vi "example_temp_monitor_multiqueue.vi"() -> ()   [LabVIEW 2025]
uses:
  <resource>/dialog/BookmarkManager/managers/Default/support/Message Queue/BMark_Message Queue.lvlib
  <resource>/dialog/BookmarkManager/managers/Default/support/User Event - Stop/BMark_User Event - Stop.lvlib
  controls_queue/UI Data.ctl
  Program Files/National Instruments/LabVIEW 2025/examples/Industry Applications/Temperature Monitoring/support/Message Queue/Temp Monitor Message Queue.lvlib
  Program Files/National Instruments/LabVIEW 2025/ProjectTemplates/Source/Core/Continuous Measurement/Logging/Logging Configuration.ctl
  Program Files/National Instruments/LabVIEW 2025/ProjectTemplates/Source/Core/Continuous Measurement/Acquisition/Signal Type.ctl
  Program Files/National Instruments/LabVIEW 2025/ProjectTemplates/Source/Core/Continuous Measurement/Acquisition/Hardware Configuration.ctl
  Program Files/National Instruments/LabVIEW 2025/ProjectTemplates/Source/Core/Continuous Measurement/Settings/Settings.ctl
panel:
  out "Do Something Ref":refnum<vi>
  out "Boolean <Replace Me>":bool
  out "Status":string
  in  "Exit":bool
  in  "Stop":bool
  in  "Settings":bool
  in  "Start":bool
  out "Data":waveform(dbl)[](graph)
  # "Continuous Measurement and Logging (NI-DAQmx)"
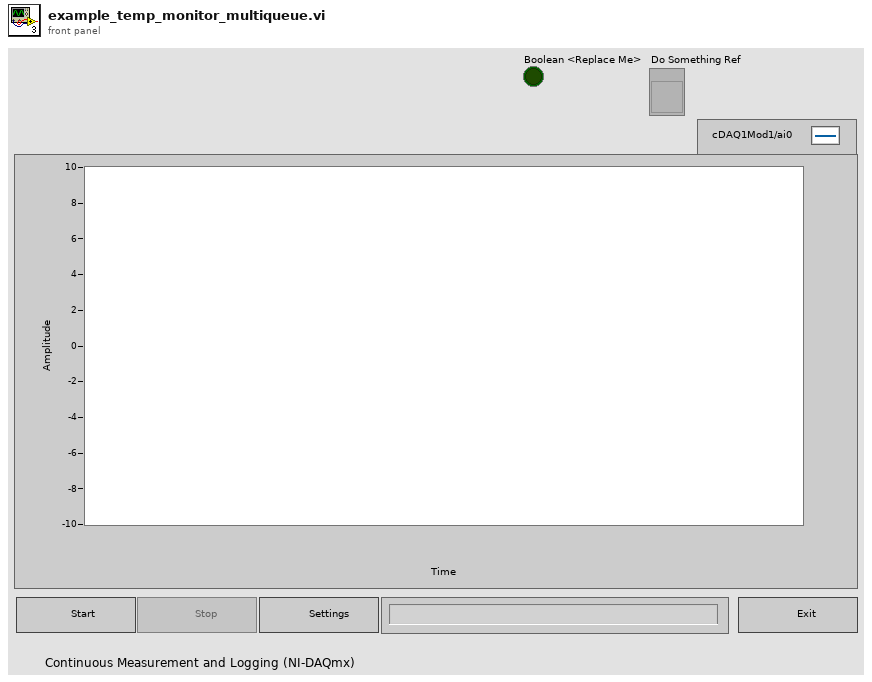
[diagram p1: front panel]
types:
  T1 = typedef "Logging.lvlib/Logging Configuration.ctl" = cluster{"Log File Base Path":path, "TDMS File Reference":refnum<k34>}
  T2 = typedef "Settings.lvlib/Settings.ctl" = cluster{"Hardware Configuration":T3, "Logging Configuration":T1}
  T3 = typedef "Acquisition.lvlib/Hardware Configuration.ctl" = cluster{"HW Refnum <Replace Me>":string, "Signal Type <Replace Me>":T4}
  T4 = typedef "Acquisition.lvlib/Signal Type.ctl" = enum16{"Sine Wave", "Square with Noise"}
  T5 = typedef "UI Data.ctl" = cluster{"Start Ref":refnum<vi>, "Stop Ref":refnum<vi>, "Settings Ref":refnum<vi>, "Exit Ref":refnum<vi>, "Status Ref":refnum<vi>, "Data Ref":refnum<vi>}
  T6 = typedef "Temp Monitor Message Queue.lvlib/All Message Queues.ctl" = cluster{"UI":refnum<queue>, "Acquisition":refnum<queue>}
  T7 = enum16{"open", "open or create", "create or replace", "create", "open (read-only)"}
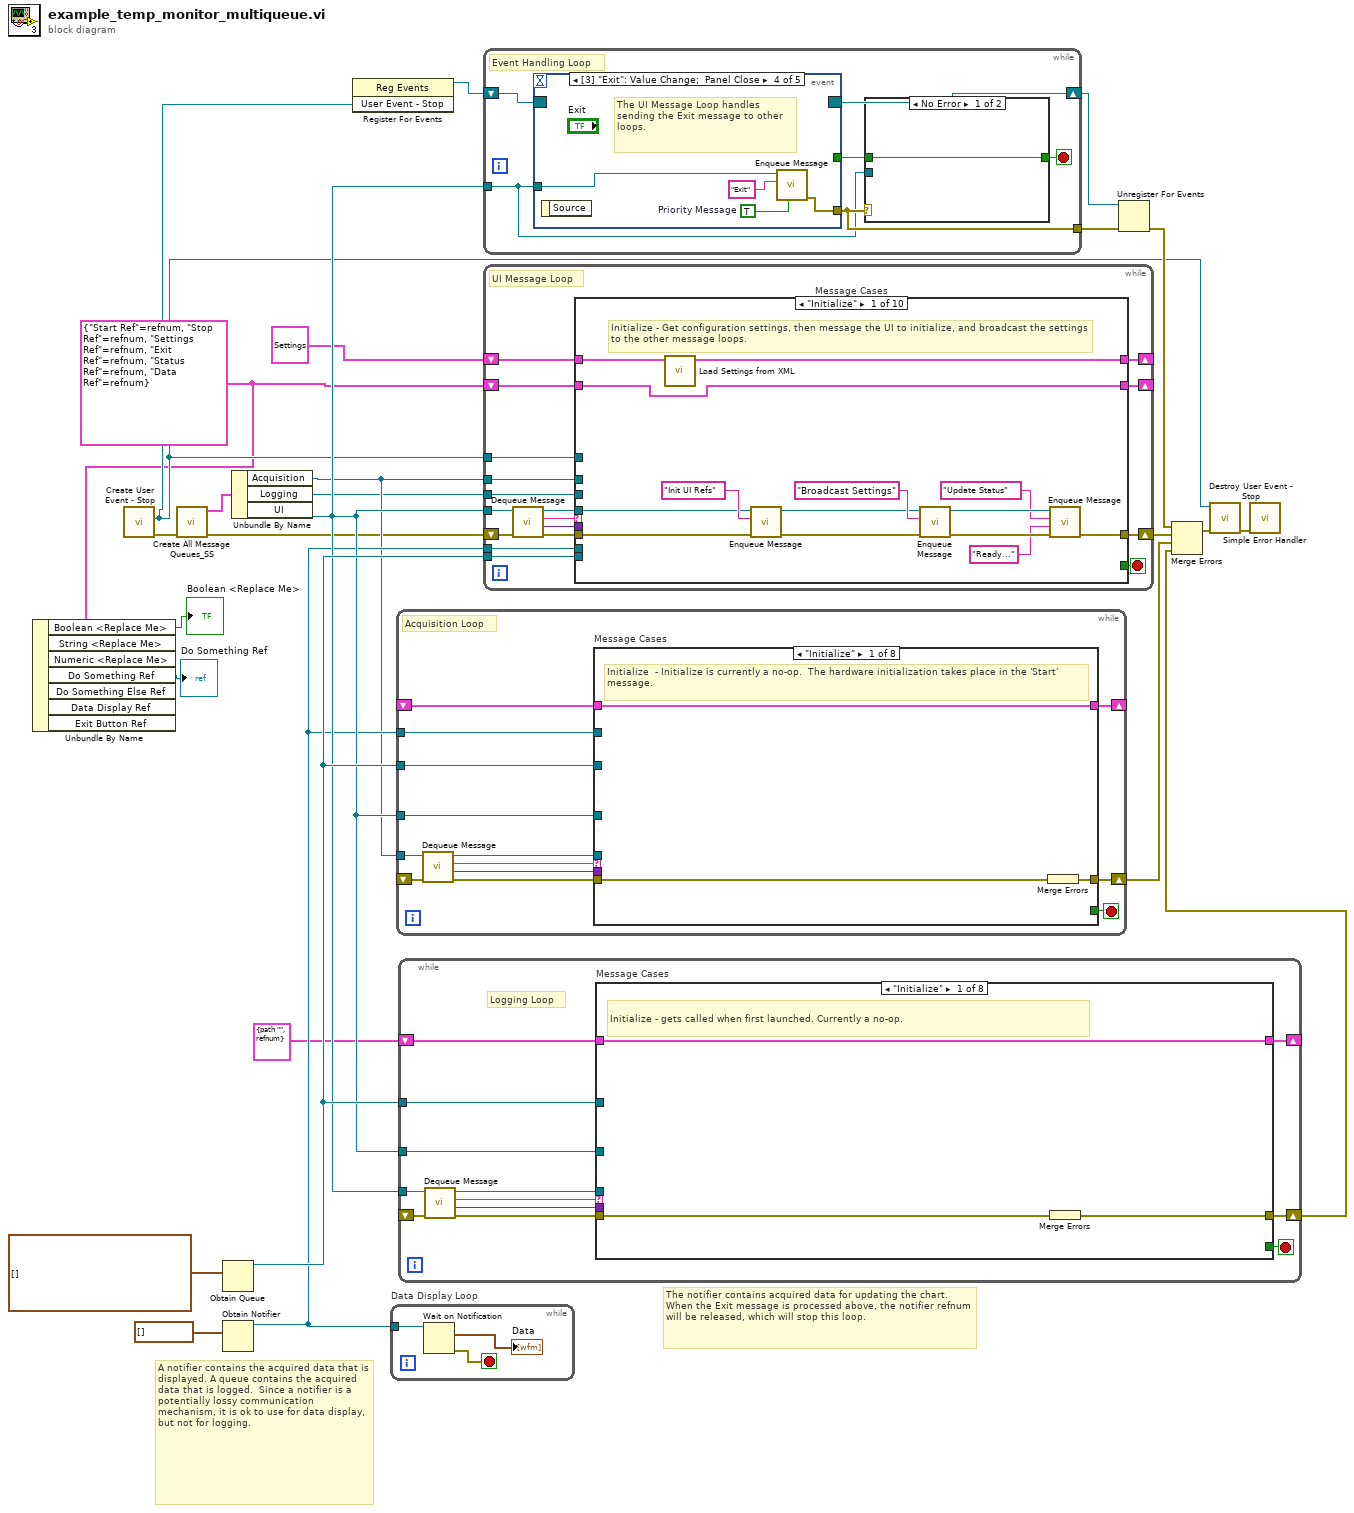
[diagram p0: block diagram]
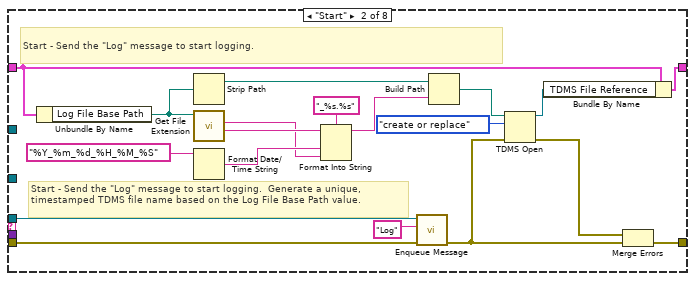
[diagram p2: hidden frame]
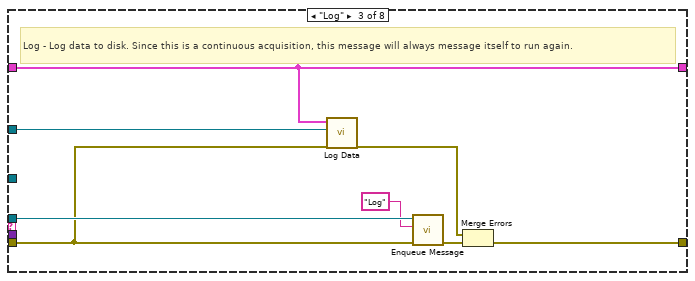
[diagram p3: hidden frame]
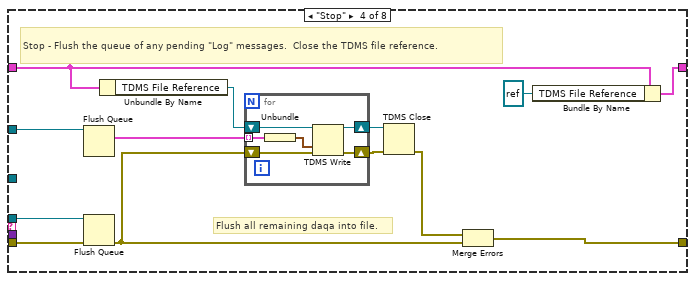
[diagram p4: hidden frame]
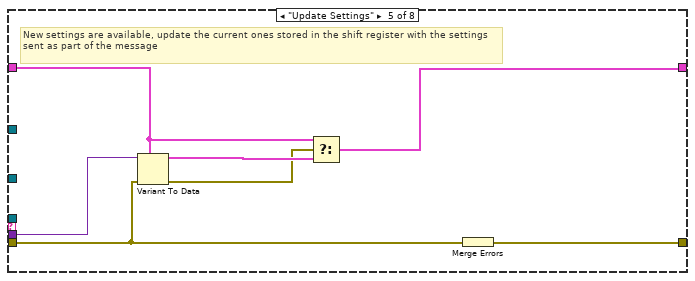
[diagram p5: hidden frame]
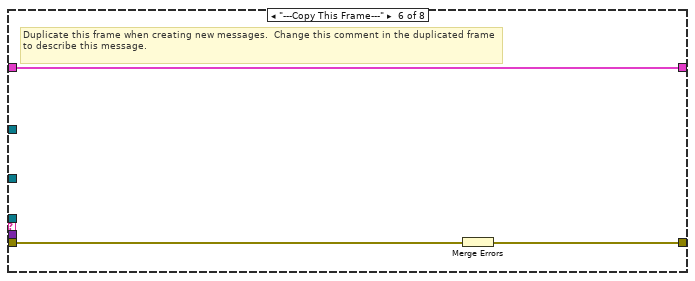
[diagram p6: hidden frame]
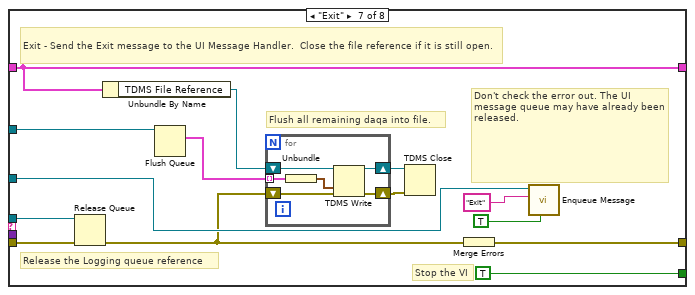
[diagram p7: hidden frame]
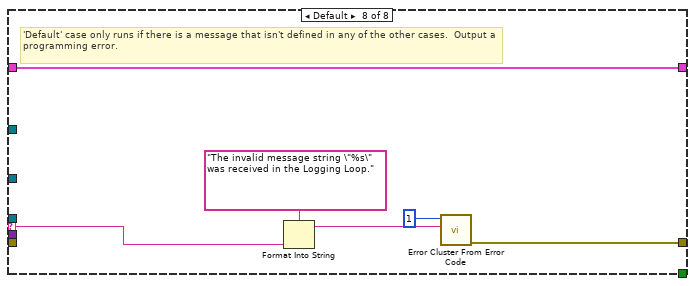
[diagram p8: hidden frame]
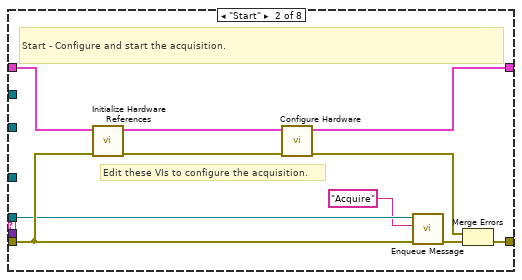
[diagram p9: hidden frame]
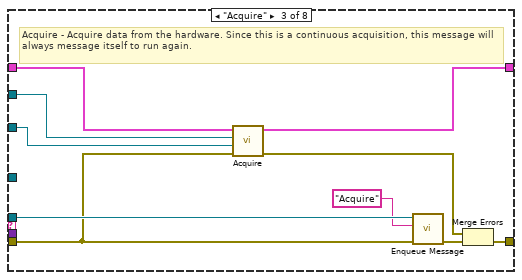
[diagram p10: hidden frame]
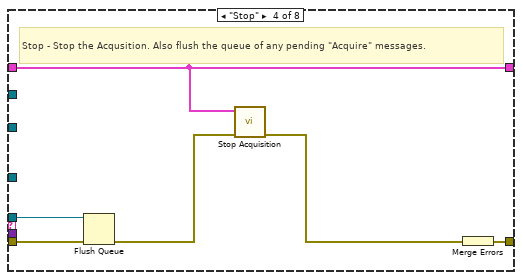
[diagram p11: hidden frame]
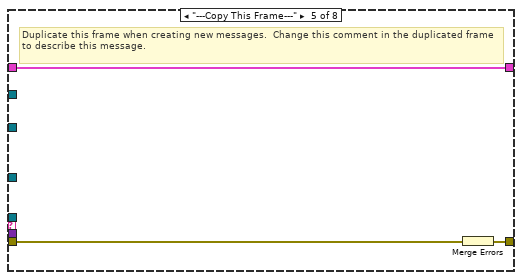
[diagram p12: hidden frame]
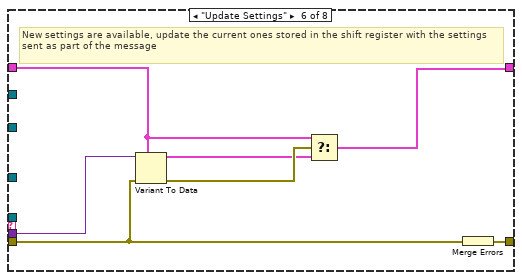
[diagram p13: hidden frame]
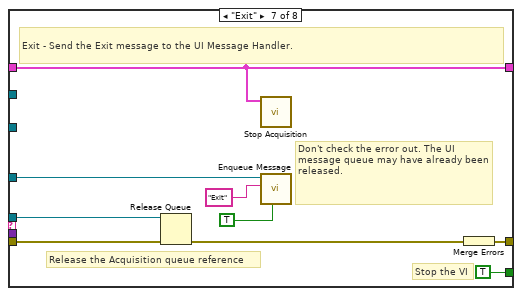
[diagram p14: hidden frame]
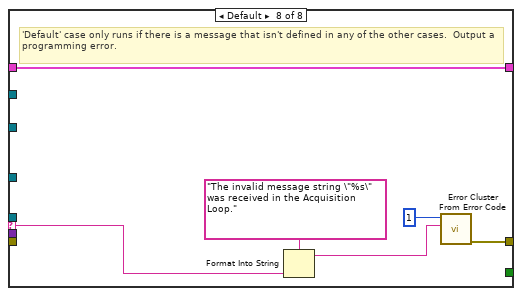
[diagram p15: hidden frame]
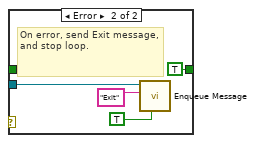
[diagram p16: hidden frame]
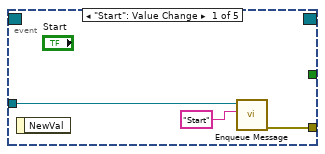
[diagram p17: hidden frame]
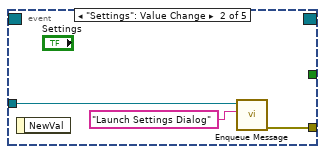
[diagram p18: hidden frame]
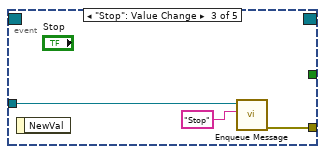
[diagram p19: hidden frame]
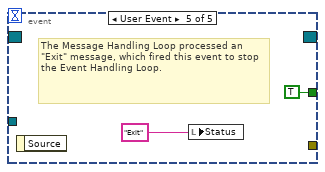
[diagram p20: hidden frame]
diagram:
  w3 = T5 {"Start Ref"=refnum, "Stop Ref"=refnum, "Settings Ref"=refnum, "Exit Ref"=refnum, "Status Ref"=refnum, "Data Ref"=refnum} ("Measurement UI Controls")
  # "A notifier contains the acquired data that is displayed. A queue contains the acquired data that is logged.  Since a notifier is a potentially lossy communication mechanism, it is ok to use for data display, but not for logging."
  # "The notifier contains acquired data for updating the chart. When the Exit message is processed above, the notifier refnum will be released, which will stop this loop."
  n1 = Unbundle By Name(w3) -> ("Boolean <Replace Me>"=→"Boolean <Replace Me>":bool, "Do Something Ref"=→"Do Something Ref":refnum<vi>)  [unwired: 5 out]
  n2 = call <resource>:"Create User Event - Stop.vi"() -> ("error out"=w9:errorcluster, "User Event - Stop"=w5:refnum<user-event>)  [unwired: 10 in]
  n3 = call "Create All Message Queues_SS.vi"("error in (no error)"=w9) -> ("error out"=w11:errorcluster, "Message Queues out"=w10:T6)  [unwired: 9 in]
  n4 = Obtain Queue(element data type=waveform(dbl)[] []) -> (queue out=w25:refnum<queue>)  [unwired: 4 in, 2 out]
  n5 = Obtain Notifier(notification data type=waveform(dbl)[] []) -> (notifier out=w23:refnum<notifier>)  [unwired: 3 in, 2 out]
  n6 = Unbundle By Name(w10) -> ("Acquisition"=w19:refnum<queue>, "Logging"=w15:refnum<queue>, "UI"=w24:refnum<queue>)
  n7 = register-events(w5) -> (reference out=w4:refnum<event-registration>)  [unwired: 2 in, 1 out]
  n8 = while "Data Display Loop" {
    tunnel: w23 -> [w28]
    stop <- w26 stop-if-true
    n9 = Wait on Notification(notifier=w28) -> (notification=→"Data":waveform(dbl)[], error out=w26:errorcluster)  [unwired: 3 in, 2 out]
  }
  n10 = while {
    tunnel: w19 -> [w32]
    shift-right: [w40] -> _
    shift-left: _ -> [w41]
    shift-right: [w38] -> w20
    shift-left: _ -> [w37]
    tunnel: w24 -> [w31]
    tunnel: w23 -> [w30]
    tunnel: w25 -> [w29]
    stop <- w39 stop-if-true
    # "Acquisition Loop"
    n11 = call <resource>:"Dequeue Message.vi"("error in (no error)"=w37, "Message Queue"=w32) -> ("error out"=w36:errorcluster, "Message Data"=w34:variant, "Message"=w35:string, "dup Message Queue"=w33:refnum<queue>)  [unwired: 6 in]
    n12 = case "Message Cases" shown="\"Initialize\"" w35 {
      selector: w35 -> [_ _ _ _ _ _ _ w93]
      tunnel: w33 -> [_ w50 w62 w65 _ _ w82 _]
      tunnel: w36 -> [w43 w52 w61 w69 w73 w74 w86 _]
      tunnel: [w44 w54 w64 w70 w71 w80 w88 w91] -> w38
      tunnel: w41 -> [w42 w53 w58 w67 w72 w76 w81 w95]
      tunnel: [w42 w46 w59 w67 w72 w75 w81 w95] -> w40
      tunnel: [_ _ _ _ _ _ TRUE _] -> w39
      tunnel: w34 -> [_ _ _ _ _ w79 _ _]
      tunnel: w31 -> [_ _ _ _ _ _ w87 _]
      tunnel: w30 -> [_ _ w56 _ _ _ _ _]
      tunnel: w29 -> [_ _ w55 _ _ _ _ _]
      frame "Initialize" {
        # "Initialize  - Initialize is currently a no-op.  The hardware initialization takes place in the 'Start' message."
        n13 = Merge Errors(w43) -> (w44:errorcluster)
      }
      frame "Start" {
        # "Edit these VIs to configure the acquisition."
        # "Start - Configure and start the acquisition."
        n14 = call "Initialize Hardware References.vi"("error in (no error)"=w52, "Hardware Resources in"=w53) -> ("error out"=w49:errorcluster, "Hardware Resources out"=w47:T3)  [unwired: 8 in]
        n15 = call "Configure Hardware.vi"("error in (no error)"=w49, "Hardware Resources in"=w47) -> ("error out"=w48:errorcluster, "Hardware Resources out"=w46:T3)  [unwired: 8 in]
        n16 = call <resource>:"Enqueue Message.vi"("error in (no error)"=w52, "Message"="Acquire", "Message Queue"=w50) -> ("error out"=w51:errorcluster)  [unwired: 7 in, 1 out]
        n17 = Merge Errors(w48, w51) -> (w54:errorcluster)
      }
      frame "Acquire" {
        # "Acquire - Acquire data from the hardware. Since this is a continuous acquisition, this message will always message itself to run again."
        n18 = call "Acquire.vi"("error in (no error)"=w61, "Data Queue"=w55, "Data Notifier"=w56, "Hardware Resources in"=w58) -> ("error out"=w60:errorcluster, "Hardware Resources out"=w59:T3)  [unwired: 6 in]
        n19 = call <resource>:"Enqueue Message.vi"("error in (no error)"=w61, "Message"="Acquire", "Message Queue"=w62) -> ("error out"=w63:errorcluster)  [unwired: 7 in, 1 out]
        n20 = Merge Errors(w60, w63) -> (w64:errorcluster)
      }
      frame "Stop" {
        # "Stop - Stop the Acqusition. Also flush the queue of any pending \"Acquire\" messages."
        n21 = Flush Queue(queue=w65, error in (no error)=w69) -> (error out=w66:errorcluster)  [unwired: 2 out]
        n22 = call "Stop Acquisition.vi"("error in (no error)"=w66, "Hardware Resources in"=w67) -> ("error out"=w68:errorcluster)  [unwired: 9 in]
        n23 = Merge Errors(w68) -> (w70:errorcluster)
      }
      frame "---Copy This Frame---" {
        # "Duplicate this frame when creating new messages.  Change this comment in the duplicated frame to describe this message."
        n24 = Merge Errors(w73) -> (w71:errorcluster)
      }
      frame "Update Settings" {
        # "New settings are available, update the current ones stored in the shift register with the settings sent as part of the message"
        n25 = Variant To Data(error in=w74, type=w76, Variant=w79) -> (data=w77:T3, error out=w78:errorcluster)
        n26 = Select(t=w76, s=w78, f=w77) -> (s? t:f=w75:T3)
        n27 = Merge Errors(w74) -> (w80:errorcluster)
      }
      frame "Exit" {
        # "Don't check the error out. The UI message queue may have already been released."
        # "Release the Acquisition queue reference"
        # "Stop the VI"
        # "Exit - Send the Exit message to the UI Message Handler."
        n28 = Release Queue(queue=w82, error in (no error)=w86) -> (error out=w83:errorcluster)  [unwired: 1 in, 2 out]
        n29 = call "Stop Acquisition.vi"("Hardware Resources in"=w81) -> ()  [unwired: 10 in, 1 out]
        n30 = call <resource>:"Enqueue Message.vi"("Priority Message? (F)"=TRUE, "Message"="Exit", "Message Queue"=w87) -> ()  [unwired: 7 in, 2 out]
        n31 = Merge Errors(w83) -> (w88:errorcluster)
      }
      frame Default {
        # "'Default' case only runs if there is a message that isn't defined in any of the other cases.  Output a programming error."
        n32 = Format Into String(format string="The invalid message string \"%s\" was received in the Acquisition Loop." ("Invalid Acquisition Message"), w93) -> (resulting string=w90:string)  [unwired: 2 in, 1 out]
        n33 = call <vilib>:"Error Cluster From Error Code.vi"("error message (\"\")"=w90, "error code (0)"=1) -> ("error out"=w91:errorcluster)  [unwired: 7 in]
      }
    }
  }
  n34 = while {
    shift-right: [w106] -> _
    shift-left: T1 {"Log File Base Path"=path "", "TDMS File Reference"=refnum} ("Logging Configuration") -> [w107]
    shift-right: [w104] -> w21
    shift-left: _ -> [w103]
    tunnel: w24 -> [w98]
    tunnel: w25 -> [w97]
    tunnel: w24 -> [w96]
    stop <- w105 stop-if-true
    # "Logging Loop"
    n35 = call <resource>:"Dequeue Message.vi"("error in (no error)"=w103, "Message Queue"=w96) -> ("error out"=w102:errorcluster, "Message Data"=w100:variant, "Message"=w101:string, "dup Message Queue"=w99:refnum<queue>)  [unwired: 6 in]
    n36 = case "Message Cases" shown="\"Initialize\"" w101 {
      selector: w101 -> [_ _ _ _ _ _ _ w190]
      tunnel: w99 -> [_ w128 w135 w148 _ _ w174 _]
      tunnel: w102 -> [w108 w126 w133 w149 w157 w166 w177 _]
      tunnel: [w110 w129 w137 w150 w163 w164 w179 w188] -> w104
      tunnel: w107 -> [w109 w117 w131 w145 w161 w165 w173 w192]
      tunnel: [w109 w114 w131 w147 w158 w165 w173 w192] -> w106
      tunnel: [_ _ _ _ _ _ TRUE _] -> w105
      tunnel: w100 -> [_ _ _ _ w162 _ _ _]
      tunnel: w98 -> [_ _ _ _ _ _ w178 _]
      tunnel: w97 -> [_ _ w130 w138 _ _ w167 _]
      frame "Initialize" {
        # "Initialize - gets called when first launched. Currently a no-op."
        n37 = Merge Errors(w108) -> (w110:errorcluster)
      }
      frame "Start" {
        # "Start - Send the \"Log\" message to start logging."
        # "Start - Send the \"Log\" message to start logging.  Generate a unique, timestamped TDMS file name based on the Log File Base Path value."
        n38 = Unbundle By Name(w117) -> ("Log File Base Path"=w124:path)
        n39 = Strip Path(path=w124) -> (stripped path=w123:path)  [unwired: 1 out]
        n40 = call <vilib>:"Get File Extension.vi"("file"=w124) -> ("filename without extension"=w122:string, "lowercase file extension"=w119:string)  [unwired: 6 in, 3 out]
        n41 = Format Date/Time String(time format string (%c)="%Y_%m_%d_%H_%M_%S") -> (date/time string=w120:string)  [unwired: 2 in]
        n42 = Format Into String(format string="_%s.%s", initial string=w122, w120, w119) -> (resulting string=w118:string)  [unwired: 1 in, 1 out]
        n43 = call <resource>:"Enqueue Message.vi"("error in (no error)"=w126, "Message"="Log", "Message Queue"=w128) -> ("error out"=w112:errorcluster)  [unwired: 7 in, 1 out]
        n44 = Build Path(base path=w123, name or relative path=w118) -> (appended path=w115:path)
        n45 = TDMS Open(8:w112, 10:T7."create or replace" ("operation (0:open)"), 11:w115) -> (0:w111:errorcluster, 3:w116:refnum<k34>)  [unwired: 4 in]
        n46 = Bundle By Name(cluster=w117, "TDMS File Reference"=w116) -> (w114:T1)
        n47 = Merge Errors(w111, w112) -> (w129:errorcluster)
      }
      frame "Log" {
        # "Log - Log data to disk. Since this is a continuous acquisition, this message will always message itself to run again."
        n48 = call "Log Data.vi"("error in (no error)"=w133, "Data Queue"=w130, "Logging Configuration"=w131) -> ("error out"=w134:errorcluster)  [unwired: 8 in]
        n49 = call <resource>:"Enqueue Message.vi"("error in (no error)"=w133, "Message"="Log", "Message Queue"=w135) -> ("error out"=w136:errorcluster)  [unwired: 7 in, 1 out]
        n50 = Merge Errors(w134, w136) -> (w137:errorcluster)
      }
      frame "Stop" {
        # "Flush all remaining daqa into file."
        # "Stop - Flush the queue of any pending \"Log\" messages.  Close the TDMS file reference."
        n51 = Flush Queue(queue=w138) -> (remaining elements=w142:cluster{waveform(dbl)[]}[])  [unwired: 1 in, 2 out]
        n52 = Flush Queue(queue=w148, error in (no error)=w149) -> (error out=w143:errorcluster)  [unwired: 2 out]
        n53 = Unbundle By Name(w145) -> ("TDMS File Reference"=w144:refnum<k34>)
        n54 = for {
          tunnel: w142 -> [w152] mode=indexing
          shift-right: [w153] -> w141
          shift-left: w144 -> [w156]
          shift-right: [w155] -> w140
          shift-left: w143 -> [w154]
          n55 = Unbundle(w152) -> (w151:waveform(dbl)[])
          n56 = TDMS Write(0:w156, 9:w151, 11:w154) -> (4:w153:refnum<k34>, 15:w155:errorcluster)  [unwired: 3 in, 2 out]
        }
        n57 = TDMS Close(8:w140, 11:w141) -> (0:w139:errorcluster)  [unwired: 1 out]
        n58 = Merge Errors(w139, w143) -> (w150:errorcluster)
        n59 = Bundle By Name(cluster=w145, "TDMS File Reference"=refnum<k34> refnum ("tdms file out")) -> (w147:T1)
      }
      frame "Update Settings" {
        # "New settings are available, update the current ones stored in the shift register with the settings sent as part of the message"
        n60 = Variant To Data(error in=w157, type=w161, Variant=w162) -> (data=w160:T1, error out=w159:errorcluster)
        n61 = Select(t=w161, s=w159, f=w160) -> (s? t:f=w158:T1)
        n62 = Merge Errors(w157) -> (w163:errorcluster)
      }
      frame "---Copy This Frame---" {
        # "Duplicate this frame when creating new messages.  Change this comment in the duplicated frame to describe this message."
        n63 = Merge Errors(w166) -> (w164:errorcluster)
      }
      frame "Exit" {
        # "Flush all remaining daqa into file."
        # "Release the Logging queue reference"
        # "Don't check the error out. The UI message queue may have already been released."
        # "Stop the VI"
        # "Exit - Send the Exit message to the UI Message Handler.  Close the file reference if it is still open."
        n64 = Release Queue(queue=w174, error in (no error)=w177) -> (error out=w169:errorcluster)  [unwired: 1 in, 2 out]
        n65 = Unbundle By Name(w173) -> ("TDMS File Reference"=w168:refnum<k34>)
        n66 = Flush Queue(queue=w167) -> (remaining elements=w170:cluster{waveform(dbl)[]}[])  [unwired: 1 in, 2 out]
        n67 = for {
          tunnel: w170 -> [w182] mode=indexing
          shift-right: [w183] -> w171
          shift-left: w168 -> [w186]
          shift-right: [w185] -> w172
          shift-left: w169 -> [w184]
          n68 = Unbundle(w182) -> (w181:waveform(dbl)[])
          n69 = TDMS Write(0:w186, 9:w181, 11:w184) -> (4:w183:refnum<k34>, 15:w185:errorcluster)  [unwired: 3 in, 2 out]
        }
        n70 = TDMS Close(8:w172, 11:w171) -> ()  [unwired: 2 out]
        n71 = Merge Errors(w169) -> (w179:errorcluster)
        n72 = call <resource>:"Enqueue Message.vi"("Priority Message? (F)"=TRUE, "Message"="Exit", "Message Queue"=w178) -> ()  [unwired: 7 in, 2 out]
      }
      frame Default {
        # "'Default' case only runs if there is a message that isn't defined in any of the other cases.  Output a programming error."
        n73 = Format Into String(format string="The invalid message string \"%s\" was received in the Logging Loop." ("Invalid Logging Message"), w190) -> (resulting string=w187:string)  [unwired: 2 in, 1 out]
        n74 = call <vilib>:"Error Cluster From Error Code.vi"("error message (\"\")"=w187, "error code (0)"=1) -> ("error out"=w188:errorcluster)  [unwired: 7 in]
      }
    }
  }
  n75 = while {
    tunnel: w24 -> [w195]
    tunnel: [w196] -> w7
    shift-right: [w194] -> w14
    shift-left: w4 -> [w193]
    stop <- w197 stop-if-true
    # "Event Handling Loop"
    n76 = event shown="[3] \"Exit\": Value Change;  Panel Close" {
      selector: w193 -> [_ _ _ _ _]
      dyn-events: [_ _ _ _ _] -> w194
      timeout: _ -> [_ _ _ _ _]
      tunnel: [_ _ _ _ TRUE ("Discard?")] -> w198
      tunnel: w195 -> [w204 w207 w211 w213 _]
      tunnel: [w206 w209 w210 w216 _] -> w196
      event "Start": Value Change {
        n77 = event-data() -> ()  [unwired: 1 in, 1 out]
        n78 = call <resource>:"Enqueue Message.vi"("Message"="Start", "Message Queue"=w204) -> ("error out"=w206:errorcluster)  [unwired: 8 in, 1 out]
      }
      event "Settings": Value Change {
        n79 = event-data() -> ()  [unwired: 1 in, 1 out]
        n80 = call <resource>:"Enqueue Message.vi"("Message"="Launch Settings Dialog", "Message Queue"=w207) -> ("error out"=w209:errorcluster)  [unwired: 8 in, 1 out]
      }
      event "Stop": Value Change {
        n81 = event-data() -> ()  [unwired: 1 in, 1 out]
        n82 = call <resource>:"Enqueue Message.vi"("Message"="Stop", "Message Queue"=w211) -> ("error out"=w210:errorcluster)  [unwired: 8 in, 1 out]
      }
      event "Exit": Value Change; Panel Close {
        w214 = TRUE  # Priority Message
        # "The UI Message Loop handles sending the Exit message to other loops."
        n83 = event-data() -> ()  [unwired: 1 in, 1 out]
        n84 = call <resource>:"Enqueue Message.vi"("Priority Message? (F)"=w214, "Message"="Exit", "Message Queue"=w213) -> ("error out"=w216:errorcluster)  [unwired: 7 in, 1 out]
      }
      event User Event {
        # "The Message Handling Loop processed an \"Exit\" message, which fired this event to stop the Event Handling Loop."
        n85 = event-data() -> ()  [unwired: 1 in, 1 out]
        n86 = local write "Status"("Exit" ("Exit String")) -> ()
      }
    }
    n87 = case shown="No Error" w196 {
      tunnel: [w199 TRUE ("Discard?")] -> w197
      tunnel: w198 -> [w199 _]
      tunnel: w195 -> [_ w200]
      frame No Error {
      }
      frame Error {
        # "On error, send Exit message, and stop loop."
        n88 = call <resource>:"Enqueue Message.vi"("Priority Message? (F)"=TRUE ("Discard?"), "Message"="Exit", "Message Queue"=w200) -> ()  [unwired: 7 in, 2 out]
      }
    }
  }
  n89 = while {
    tunnel: w24 -> [w227]
    tunnel: w5 -> [w233]
    shift-right: [w234] -> w6
    shift-left: w11 -> [w232]
    shift-right: [w226] -> _
    shift-left: T2 {"Hardware Configuration"={"HW Refnum <Replace Me>"="", "Signal Type <Replace Me>"=enum."Sine Wave"}, "Logging Configuration"={"Log File Base Path"=path "", "TDMS File Reference"=refnum}} ("Settings") -> [w225]
    shift-right: [w223] -> _
    shift-left: w3 -> [w224]
    tunnel: w19 -> [w222]
    tunnel: w15 -> [w221]
    tunnel: w23 -> [w220]
    tunnel: w25 -> [w219]
    stop <- w235 stop-if-true
    # "UI Message Loop"
    n90 = call <resource>:"Dequeue Message.vi"("error in (no error)"=w232, "Message Queue"=w227) -> ("error out"=w231:errorcluster, "Message Data"=w229:variant, "Message"=w230:string, "dup Message Queue"=w228:refnum<queue>)  [unwired: 6 in]
    n91 = case "Message Cases" shown="\"Initialize\"" w230 {
      selector: w230 -> [_ _ _ _ _ _ _ _ _ w367]
      tunnel: w228 -> [w239 _ _ w294 w316 _ w333 w347 _ _]
      tunnel: w231 -> [w238 w264 w271 w293 w315 w322 w335 w355 w361 _]
      tunnel: [w245 w264 w272 w295 w317 w328 w330 w356 w360 w365] -> w234
      tunnel: [_ _ _ _ _ _ _ TRUE _ _] -> w235
      tunnel: w229 -> [_ _ w270 _ _ _ _ _ _ _]
      tunnel: w233 -> [_ _ _ _ _ _ _ w354 _ _]
      tunnel: [w248 w263 w266 w292 w314 w326 w332 w352 w359 w363] -> w226
      tunnel: w225 -> [w249 w263 w266 w292 w314 w326 w336 w352 w359 w363]
      tunnel: w224 -> [w241 w262 w265 w289 w298 w320 w329 w350 w358 w362]
      tunnel: [w241 w259 w265 w289 w298 w320 w329 w350 w358 w362] -> w223
      tunnel: w222 -> [_ _ _ w275 w301 w319 _ w349 _ _]
      tunnel: w221 -> [_ _ _ w278 w304 w318 _ w348 _ _]
      tunnel: w220 -> [_ _ _ _ _ _ _ w346 _ _]
      tunnel: w219 -> [_ _ _ _ _ _ _ w342 _ _]
      frame "Initialize" {
        # "Initialize - Get configuration settings, then message the UI to initialize, and broadcast the settings to the other message loops."
        n92 = call "Load Settings from XML.vi"("Settings in"=w249) -> ("Settings out"=w248:T2)  [unwired: 9 in, 1 out]
        n93 = call <resource>:"Enqueue Message.vi"("error in (no error)"=w238, "Message"="Init UI Refs", "Message Queue"=w239) -> ("error out"=w236:errorcluster, "dup Message Queue"=w237:refnum<queue>)  [unwired: 7 in]
        n94 = call <resource>:"Enqueue Message.vi"("error in (no error)"=w236, "Message"="Broadcast Settings", "Message Queue"=w237) -> ("error out"=w247:errorcluster, "dup Message Queue"=w246:refnum<queue>)  [unwired: 7 in]
        n95 = call <resource>:"Enqueue Message.vi"("error in (no error)"=w247, "Message Data"="Ready..." ("Ready..."), "Message"="Update Status", "Message Queue"=w246) -> ("error out"=w245:errorcluster)  [unwired: 6 in, 1 out]
      }
      frame "Init UI Refs" {
        # "Enable: Start, Exit, Settings\nDisable: Stop"
        # "Init UI Refs - Store control references for UI controls.  Also enable/disable controls appropriately."
        n96 = control-ref of="Start"() -> (w253:refnum<vi>)
        n97 = control-ref of="Data"() -> (w260:refnum<vi>)
        n98 = property class="Bool" props=["Value"]() -> ()  [unwired: 2 in, 3 out]
        n99 = control-ref of="Stop"() -> (w254:refnum<vi>)
        n100 = control-ref of="Settings"() -> (w252:refnum<vi>)
        n101 = control-ref of="Exit"() -> (w251:refnum<vi>)
        n102 = control-ref of="Status"() -> (w261:refnum<vi>)
        n103 = Bundle By Name(cluster=w262, "Boolean <Replace Me>"=w253, "String <Replace Me>"=w254, "Numeric <Replace Me>"=w252, "Do Something Ref"=w251, "Do Something Else Ref"=w261, "Data Display Ref"=w260) -> (w259:T5)
        n104 = property class="VI"("Front Panel.Closeable"=TRUE ("Front Panel Window:Closeable")) -> ()  [unwired: 2 in, 2 out]
        n105 = Build Array(w253, w252, w251) -> (w257:refnum<vi>[])
        n106 = Build Array(w254) -> (w256:refnum<vi>[])
        n107 = call "Set Enable State on Multiple Controls.vi"("Enable?"=TRUE, "Controls"=w257) -> ()  [unwired: 10 in]
        n108 = call "Set Enable State on Multiple Controls.vi"("Enable?"=FALSE, "Controls"=w256) -> ()  [unwired: 10 in]
      }
      frame "Update Status" {
        # "Update Display - Convert the message data to a string to display in the Status indicator."
        n109 = Variant To Data(error in=w271, type="", Variant=w270) -> (data=→"Status":string, error out=w268:errorcluster)
        n110 = Merge Errors(w268) -> (w272:errorcluster)
      }
      frame "Start" {
        # "Message Acquisition and Logging loops to start"
        # "Enable: Stop\nDisable: Start, Exit, Settings"
        # "Start - Enable/Disable buttons appropriately for an acquisition that has started, and update status display."
        n111 = Unbundle By Name(w289) -> ("String <Replace Me>"=w284:string, "Boolean <Replace Me>"=w283:bool, "Do Something Ref"=w282:refnum<vi>, "Numeric <Replace Me>"=w281:dbl)
        n112 = call <resource>:"Enqueue Message.vi"("error in (no error)"=w293, "Message Data"="Acquiring and Logging..." ("Acquiring and Logging..."), "Message"="Update Status", "Message Queue"=w294) -> ("error out"=w280:errorcluster)  [unwired: 6 in, 1 out]
        n113 = Build Array(w283, w282, w281) -> (w287:bool[])
        n114 = Build Array(w284) -> (w286:string[])
        n115 = call "Set Enable State on Multiple Controls.vi"("Enable?"=TRUE, "Controls"=w286) -> ()  [unwired: 10 in]
        n116 = call "Set Enable State on Multiple Controls.vi"("Enable?"=FALSE, "Controls"=w287) -> ()  [unwired: 10 in]
        n117 = call <resource>:"Enqueue Message.vi"("error in (no error)"=w280, "Message"="Start", "Message Queue"=w278) -> ("error out"=w277:errorcluster)  [unwired: 7 in, 1 out]
        n118 = call <resource>:"Enqueue Message.vi"("error in (no error)"=w277, "Message"="Start", "Message Queue"=w275) -> ("error out"=w276:errorcluster)  [unwired: 7 in, 1 out]
        n119 = property class="VI"("Front Panel.Closeable"=FALSE ("Front Panel Window:Closeable")) -> ()  [unwired: 2 in, 2 out]
        n120 = Merge Errors(w276) -> (w295:errorcluster)
      }
      frame "Stop" {
        # "Message Acquisition and Logging loops to stop"
        # "Enable: Start, Exit, Settings\nDisable: Stop"
        # "Stop - Enable/Disable buttons appropriately for an acquisition that has stopped, and update status display."
        n121 = Unbundle By Name(w298) -> ("String <Replace Me>"=w307:string)  [unwired: 3 out]
        n122 = control-ref of="Do Something Ref"() -> (w296:refnum<vi>)
        n123 = control-ref of="Boolean <Replace Me>"() -> (w297:refnum<vi>)
        n124 = call <resource>:"Enqueue Message.vi"("error in (no error)"=w315, "Message Data"="Ready..." ("Ready..."), "Message"="Update Status", "Message Queue"=w316) -> ("error out"=w306:errorcluster)  [unwired: 6 in, 1 out]
        n125 = Build Array(w297, w296) -> (w310:refnum<vi>[])  [unwired: 1 in]
        n126 = Build Array(w307) -> (w309:string[])
        n127 = call "Set Enable State on Multiple Controls.vi"("Enable?"=FALSE, "Controls"=w309) -> ()  [unwired: 10 in]
        n128 = call "Set Enable State on Multiple Controls.vi"("Enable?"=TRUE, "Controls"=w310) -> ()  [unwired: 10 in]
        n129 = call <resource>:"Enqueue Message.vi"("error in (no error)"=w306, "Message"="Stop", "Message Queue"=w304) -> ("error out"=w303:errorcluster)  [unwired: 7 in, 1 out]
        n130 = property class="VI"("Front Panel.Closeable"=TRUE ("Front Panel Window:Closeable")) -> ()  [unwired: 2 in, 2 out]
        n131 = call <resource>:"Enqueue Message.vi"("error in (no error)"=w303, "Message"="Stop", "Message Queue"=w301) -> ("error out"=w302:errorcluster)  [unwired: 7 in, 1 out]
        n132 = Merge Errors(w302) -> (w317:errorcluster)
      }
      frame "Broadcast settings" {
        w321 = "Update Settings" ("Message")
        # "Send the 'Update Settings' message to the Logging and Acqusition message loops."
        n133 = Unbundle By Name(w326) -> ("Hardware Configuration"=w325:T3, "Logging Configuration"=w324:T1)
        n134 = call <resource>:"Enqueue Message.vi"("Message Data"=w325, "Message"=w321, "Message Queue"=w319) -> ("error out"=w327:errorcluster)  [unwired: 7 in, 1 out]
        n135 = call <resource>:"Enqueue Message.vi"("error in (no error)"=w327, "Message Data"=w324, "Message"=w321, "Message Queue"=w318) -> ("error out"=w323:errorcluster)  [unwired: 6 in, 1 out]
        n136 = Merge Errors(w323, w322) -> (w328:errorcluster)
      }
      frame "Launch Settings Dialog" {
        # "Launch the Settings Dialog when the user clicks the 'Settings' button."
        n137 = call "Settings Dialog.vi"("error in (no error)"=w335, "Settings in"=w336) -> ("error out"=w331:errorcluster, "Cancelled?"=w334:bool, "Settings out"=w332:T2)  [unwired: 6 in, 1 out]
        n138 = case shown="False" w334 {
          tunnel: w333 -> [w340 _]
          tunnel: w331 -> [w339 w341]
          tunnel: [w338 w341] -> w330
          frame False {
            n139 = call <resource>:"Enqueue Message.vi"("error in (no error)"=w339, "Message"="Broadcast Settings", "Message Queue"=w340) -> ("error out"=w338:errorcluster)  [unwired: 7 in, 1 out]
          }
          frame True {
          }
        }
      }
      frame "Exit" {
        w351 = "Exit" ("Message")
        # "Don't check the error outs. The acquisition and logging queues may have already been released."
        # "Close references owned by the Main VI."
        # "Stop the VI"
        # "Exit - Fire the User Event to stop the Event Handling Loop.  Also send Exit messages to the Acqusition and Logging loops."
        n140 = Release Queue(queue=w347, error in (no error)=w355) -> (error out=w345:errorcluster)  [unwired: 1 in, 2 out]
        n141 = call <resource>:"Fire User Event - Stop.vi"("User Event - Stop"=w354) -> ("error out"=w353:errorcluster)  [unwired: 10 in]
        n142 = Release Notifier(notifier=w346, error in (no error)=w345) -> (error out=w344:errorcluster)  [unwired: 1 in, 2 out]
        n143 = Release Queue(queue=w342, error in (no error)=w344) -> (error out=w343:errorcluster)  [unwired: 1 in, 2 out]
        n144 = call <resource>:"Enqueue Message.vi"("Message"=w351, "Message Queue"=w349) -> ()  [unwired: 8 in, 2 out]
        n145 = call <resource>:"Enqueue Message.vi"("Message"=w351, "Message Queue"=w348) -> ()  [unwired: 8 in, 2 out]
        n146 = Merge Errors(w353, w343) -> (w356:errorcluster)
      }
      frame "---Copy This Frame---" {
        # "Duplicate this frame when creating new messages.  Change this comment in the duplicated frame to describe this message."
        n147 = Merge Errors(w361) -> (w360:errorcluster)
      }
      frame Default {
        # "'Default' case only runs if there is a message that isn't defined in any of the other cases.  Output a programming error."
        n148 = Format Into String(format string="The invalid message string \"%s\" was received in the Message Handling Loop." ("Invalid Message Loop Message"), w367) -> (resulting string=w364:string)  [unwired: 2 in, 1 out]
        n149 = call <vilib>:"Error Cluster From Error Code.vi"("error message (\"\")"=w364, "error code (0)"=1) -> ("error out"=w365:errorcluster)  [unwired: 7 in]
      }
    }
  }
  n150 = Unregister For Events(event registration refnum=w14, error in=w7) -> (error out=w13:errorcluster)
  n151 = Merge Errors(w13, w6, w20, w21) -> (w8:errorcluster)
  n152 = call <resource>:"Destroy User Event - Stop.vi"("error in (no error)"=w8, "User Event - Stop"=w5) -> ("error out"=w17:errorcluster)  [unwired: 9 in]
  n153 = call <vilib>:"Simple Error Handler.vi"("error in (no error)"=w17) -> ()  [unwired: 4 in, 5 out]
